vi "Set mode (M).vi"(8 "Error In":errorcluster, 10 "Mode":u8(ring) items=["0", "1"], 11 "VISA resource name in":refnum<visa-resource-name>) -> (0 "Error out":errorcluster, 1 "ACK":bool, 2 "L_data":u16, 3 "VISA resource name out":refnum<visa-resource-name>)   [LabVIEW 2015]
uses:
  Ctls/Cmd str.ctl
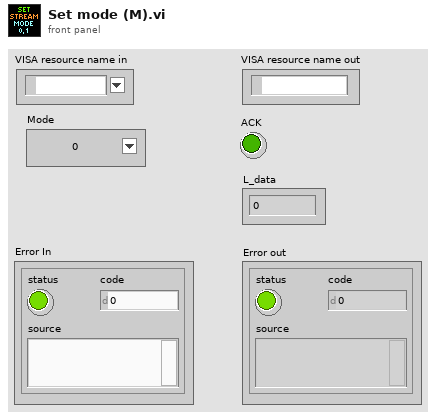
[diagram p1: front panel]
types:
  T1 = typedef "Cmd str.ctl" = string
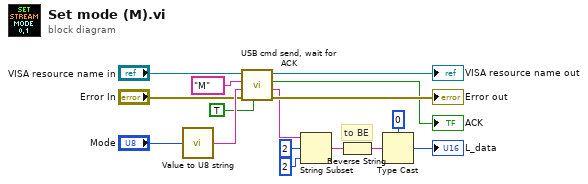
[diagram p0: block diagram]
diagram:
  # "to BE"
  n1 = call "Value to U8 string.vi"("Value"="Mode") -> ("U8 str"=w16:string)
  n2 = call "USB cmd send, wait for ACK.vi"("Wait for ACK?"=TRUE, "Error In"="Error In", "4 byte config str"=w16, "Cmd"=T1 "M", "VISA resource name in"="VISA resource name in") -> ("Error out"=→"Error out":errorcluster, "Return msg"=w7:string, "ACK ok"=→"ACK":bool, "VISA resource name out"=→"VISA resource name out":refnum<visa-resource-name>)  [unwired: 1 in]
  n3 = String Subset(string=w7, offset (0)=2, length (rest)=2 ("length (rest)")) -> (substring=w4:string)
  n4 = Reverse String(1:w4) -> (0:w1:string)
  n5 = Type Cast(type=u16 0 ("offset (0)"), x=w1) -> (*(type *) &x=→"L_data":u16)
